vi "reflectionExample.vi"() -> ()   [LabVIEW 2020]
uses:
  D2/D2.lvclass
  D1/D1.lvclass
  D/D.lvclass
  C/C.lvclass
  B2/B2.lvclass
  B1/B1.lvclass
  B/B.lvclass
  A/A.lvclass
  Reflection/reflectionPool.vi
  Reflection/Reflection.lvclass
panel:
  in  "Stop":bool
  in  "Selected Class":i32(listbox)
  in  "A.lvclass":refnum<class "A.lvclass">
  in  "B.lvclass":refnum<class "B.lvclass">
  in  "B1.lvclass":refnum<class "B1.lvclass">
  in  "B2.lvclass":refnum<class "B2.lvclass">
  in  "C.lvclass":refnum<class "C.lvclass">
  in  "D.lvclass":refnum<class "D.lvclass">
  in  "D1.lvclass":refnum<class "D1.lvclass">
  in  "D2.lvclass":refnum<class "D2.lvclass">
  out "Hierarchy of Selected Class":i32(listbox)
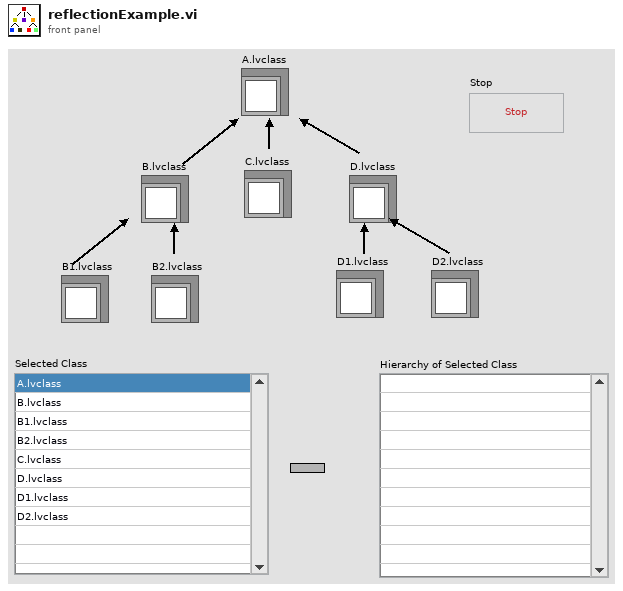
[diagram p1: front panel]
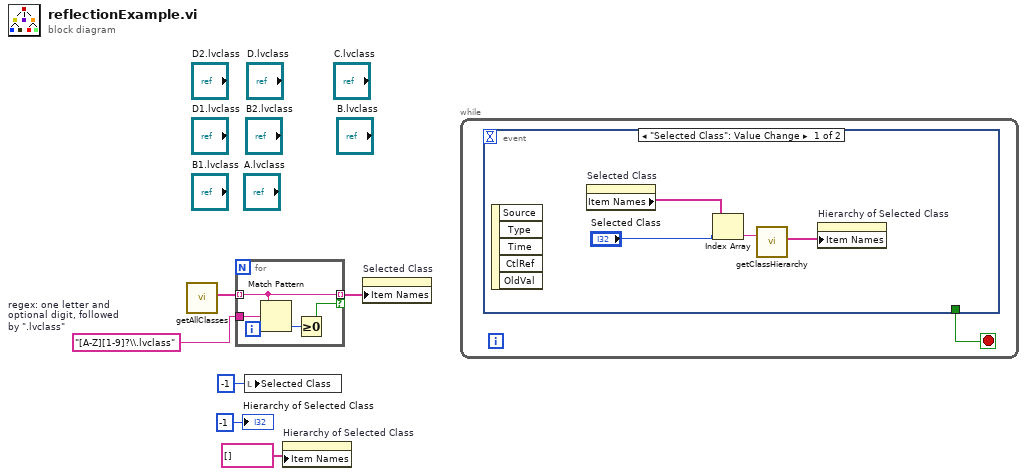
[diagram p0: block diagram]
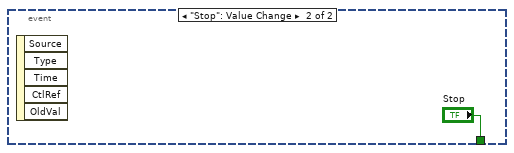
[diagram p2: hidden frame]
diagram:
  w2 = "[A-Z][1-9]?\\.lvclass"  # regex: one letter and optional digit, followed by ".lvclass"
  n1 = call "getAllClasses.vi"() -> ("all classes"=w3:string[])  [unwired: 10 in, 1 out]
  n2 = for {
    tunnel: [w10] -> w4 mode=indexing if=w7
    tunnel: w3 -> [w10] mode=indexing
    tunnel: w2 -> [w9]
    n3 = Match Pattern(string=w10, regular expression=w9) -> (offset past match=w8:i32)  [unwired: 1 in, 3 out]
    n4 = Greater Or Equal To 0?(x=w8) -> (x >= 0?=w7:bool)
  }
  n5 = local write "Selected Class"(-1 ("Selected Class")) -> ()
  n6 = property on="Hierarchy of Selected Class" class="LstBox (strict)"("Item Names"=string[] []) -> ()  [unwired: 2 in, 2 out]
  n7 = property on="Selected Class" class="LstBox (strict)"("Item Names"=w4) -> ()  [unwired: 2 in, 2 out]
  n8 = while {
    stop <- w11 stop-if-true
    n9 = event shown="[0] \"Selected Class\": Value Change" {
      selector: _ -> [_ _]
      dyn-events: _ -> [_ _]
      timeout: _ -> [_ _]
      tunnel: [_ "Stop"] -> w11
      event "Selected Class": Value Change {
        n10 = event-data() -> ()  [unwired: 1 in, 5 out]
        n11 = property on="Selected Class" class="LstBox (strict)"() -> ("Item Names"=w14:string[])  [unwired: 2 in, 2 out]
        n12 = Index Array(array=w14, index="Selected Class") -> (element=w13:string)
        n13 = call "getClassHierarchy.vi"("className"=w13) -> ("classHierarchy"=w12:string[])  [unwired: 9 in, 1 out]
        n14 = property on="Hierarchy of Selected Class" class="LstBox (strict)"("Item Names"=w12) -> ()  [unwired: 2 in, 2 out]
      }
      event "Stop": Value Change {
        n15 = event-data() -> ()  [unwired: 1 in, 5 out]
      }
    }
  }
  "Hierarchy of Selected Class" <- -1 ("Hierarchy of Selected Class")
